vi "Save 1 Set Of Data Test.vi"() -> ()   [LabVIEW 2012]
uses:
  TypeDef/WeatherData.ctl
  <vilib>/httpClient/LabVIEWHTTPClient.lvlib
  <vilib>/addons/database/NI_Database_API.lvlib
  <vilib>/addons/database/Connection.llb/DB Tools Open Connec (Path).vi
panel:
  in  "Time Stamp":timestamp
  in  "Airport Code":string
  out "Result Data Array":T1[](array[typedef])
  out "DB Call Error":errorcluster
  out "Web Call Error":errorcluster
  in  "password":string="password123%%%"
  in  "userID":string="john"
  in  "connection information":path
  out "body":string
  out "headers":string
  out "url":string="http://www.wunderground.com/history/airport/KROC/2013/11/24/DailyHistory.html?format=1"
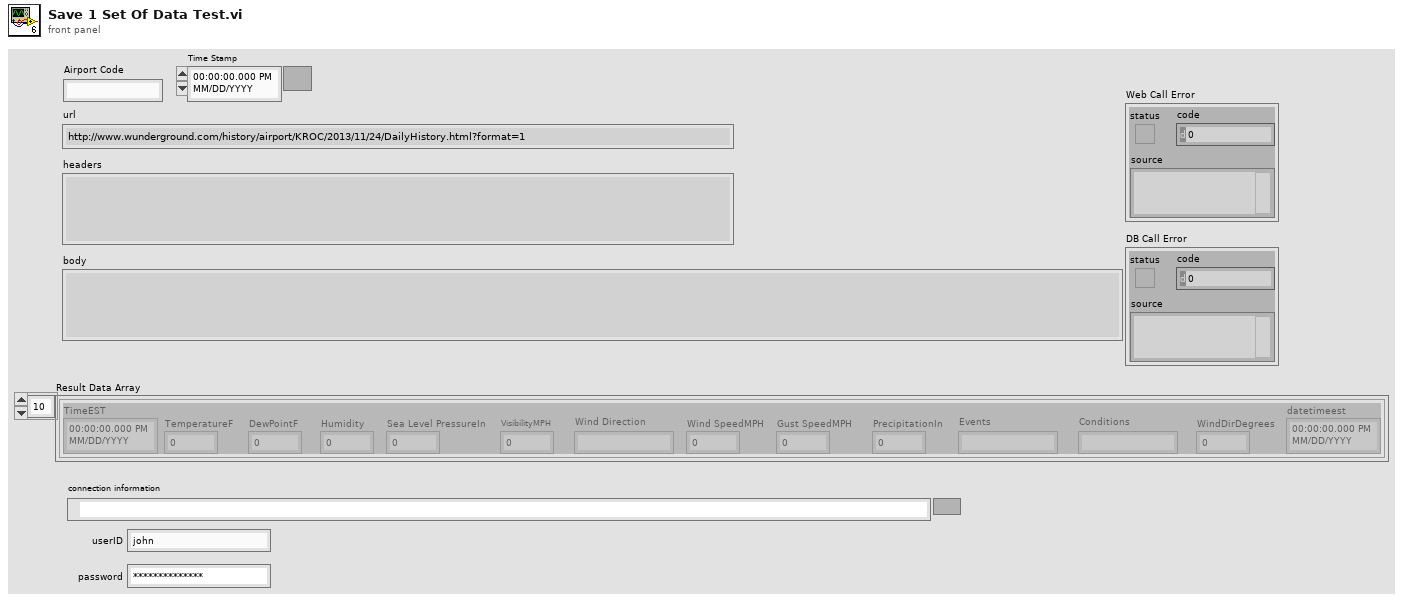
[diagram p1: front panel]
types:
  T1 = typedef "WeatherData.ctl" = cluster{"TimeEST":timestamp, "TemperatureF":dbl, "DewPointF":dbl, "Humidity":i32, "Sea Level PressureIn":dbl, "VisibilityMPH":dbl, "Wind Direction":string, "Wind SpeedMPH":dbl, "Gust SpeedMPH":dbl, "PrecipitationIn":dbl, "Events":string, "Conditions":string, "WindDirDegrees":i32, "datetimeest":timestamp}
  T2 = typedef "LabVIEWHTTPClient.lvlib/ClientHandle.ctl" = refnum<k1>
  T3 = typedef "NI_Database_API.lvlib/Conn ObjectReference.ctl" = refnum<k1>
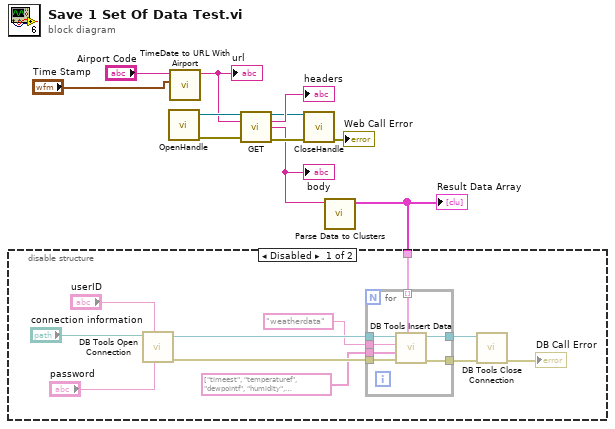
[diagram p0: block diagram]
diagram:
  n1 = call <vilib>:"OpenHandle.vi"() -> ("client handle out"=w11:T2, "error out"=w10:errorcluster)  [unwired: 14 in]
  n2 = call "TimeDate to URL With Airport.vi"("Time Stamp"="Time Stamp", "Airport Code"="Airport Code") -> ("URL"=w3:string)  [unwired: 9 in]
  "url" <- w3
  n3 = call <vilib>:"GET.vi"("client handle"=w11, "url"=w3, "error in (no error)"=w10) -> ("client handle out"=w8:T2, "headers"=→"headers":string, "body"=w6:string, "error out"=w7:errorcluster)  [unwired: 9 in]
  "body" <- w6
  n4 = call <vilib>:"CloseHandle.vi"("client handle"=w8, "error in (no error)"=w7) -> ("error out"=→"Web Call Error":errorcluster)  [unwired: 13 in]
  n5 = call "Parse Data to Clusters.vi"("body Text"=w6) -> ("Result Data Array"=w5:T1[])  [unwired: 10 in]
  "Result Data Array" <- w5
  n6 = disable-structure shown="Disabled" {
    disable-tunnel: w5 -> [w13 _]
    frame Disabled {
      n7 = call-poly <vilib>:"DB Tools Open Connection.vi"("password"="password", "userID"="userID", "connection information"="connection information") -> ("error out"=w18:errorcluster, "connection reference"=w19:T3)  [unwired: 5 in]
      n8 = for {
        tunnel: w19 -> [w29]
        tunnel: w18 -> [w28]
        tunnel: string[] ["timeest", "temperaturef", "dewpointf", "humidity", "sealevelpressurein", "visibilitymph", "winddirection", "windspeedmph", "gustspeedmph", "precipitationin", "events", "conditions", "winddirdegrees", "datetimeest"] ("subarray 3") -> [w27]
        tunnel: "weatherdata" ("table") -> [w26]
        tunnel: [w25] -> w15
        tunnel: [w24] -> w14
        tunnel: w13 -> [w23] mode=indexing
        n9 = call <vilib>:"DB Tools Insert Data.vi"("data"=w23, "error in (no error)"=w28, "columns"=w27, "table"=w26, "connection reference"=w29) -> ("error out"=w25:errorcluster, "connection reference out"=w24:T3)  [unwired: 5 in]
      }
      n10 = call <vilib>:"DB Tools Close Connection.vi"("error in (no error)"=w15, "connection reference"=w14) -> ("error out"=→"DB Call Error":errorcluster)  [unwired: 5 in]
    }
    frame Enabled {
    }
  }
